vi "Process Thrust.vi"(11 "Arilou in":refnum<class "Arilou.lvclass">) -> (3 "Arilou out":refnum<class "Arilou.lvclass">)   [LabVIEW 2021, in "Arilou.lvclass"]
uses:
  Arilou.lvclass
  Element/Element.lvclass
  Motion/Motion.lvclass
  Re-use Libraries/Vector 2D/Vector 2D.lvclass
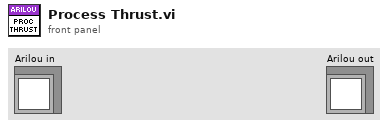
[diagram p1: front panel]
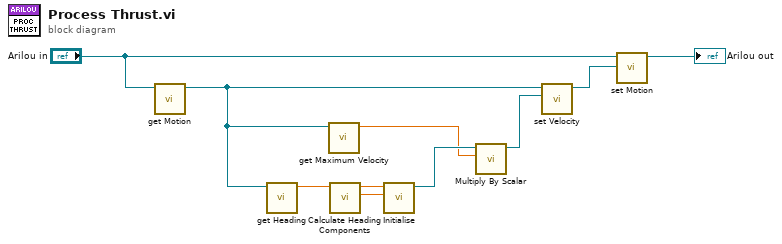
[diagram p0: block diagram]
diagram:
  n1 = call "get Motion.vi"("Element in"="Arilou in") -> ("Motion"=w5:refnum<class "Motion.lvclass">)  [unwired: 10 in]
  n2 = call "get Heading.vi"("Motion in"=w5) -> ("Heading [deg]"=w8:sgl)  [unwired: 10 in]
  n3 = call "get Maximum Velocity.vi"("Motion in"=w5) -> ("Maximum Velocity"=w1:sgl)  [unwired: 10 in]
  n4 = call "Calculate Heading Components.vi"("Heading In [deg]"=w8) -> ("Sin Heading"=w3:sgl, "Cos Heading"=w4:sgl)  [unwired: 9 in]
  n5 = call "Initialise.vi"("y"=w3, "x"=w4) -> ("Vector 2D out"=w2:refnum<class "Vector 2D.lvclass">)  [unwired: 9 in]
  n6 = call "Multiply By Scalar.vi"("x"=w1, "A"=w2) -> ("Ax"=w6:refnum<class "Vector 2D.lvclass">)  [unwired: 9 in]
  n7 = call "set Velocity.vi"("Velocity"=w6, "Motion in"=w5) -> ("Motion out"=w7:refnum<class "Motion.lvclass">)  [unwired: 9 in]
  n8 = call "set Motion.vi"("Motion"=w7, "Element in"="Arilou in") -> ("Element out"=→"Arilou out":refnum<class "Arilou.lvclass">)  [unwired: 9 in]
